vi "Excel_Read.vi"(6 "Cell to Read":string="C2", 7 "Worksheet Number":i32=1, 8 "error in (no error)":errorcluster, 9 "Sheets Reference In":refnum<k7>) -> (0 "error out":errorcluster, 1 "Sheets Reference Out":refnum<k7>, 4 "Result":dbl=6.0)   [LabVIEW 2014]
doc: "This VI demonstrates the use of ActiveX to write a table into a Microsoft Excel worksheet."
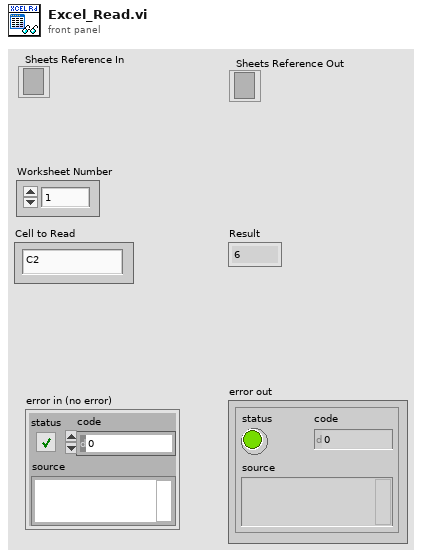
[diagram p1: front panel]
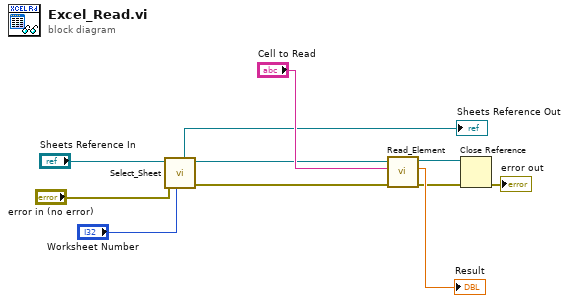
[diagram p0: block diagram]
diagram:
  n1 = call "Select_Sheet.vi"("Worksheet Number"="Worksheet Number", "error in (no error)"="error in (no error)", "Automation Refnum in"="Sheets Reference In") -> ("error out"=w3:errorcluster, "Automation Refnum out"=w4:refnum<k7>, "Sheets Refnum"=→"Sheets Reference Out":refnum<k7>)  [unwired: 6 in]
  n2 = call "Read_Element.vi"("error in (no error)"=w3, "Cell to Read"="Cell to Read", "Automation Refnum in"=w4) -> ("error out"=w7:errorcluster, "Result"=→"Result":dbl, "reference out"=w8:refnum<k7>)  [unwired: 6 in]
  n3 = Close Reference(reference=w8, error in (no error)=w7) -> (error out=→"error out":errorcluster)
